vi "setControlAmplitude.vi"(8 "error in":errorcluster, 9 "amplitude":i32, 10 "axis":i32, 11 "connection ID":i32) -> (0 "error out":errorcluster, 2 "axis_out":i32, 3 "connection ID":i32)   [LabVIEW 2016]
doc: "This function sets the amplitude of the actuator signal of the selected axis."
panel:
  out "params_cluster":cluster{"axis":i32, "amplitude":i32}
  in  "Params_cluster":cluster{"integer":i32, "integer":i32}
  in  "results_cluster":cluster{"errNo":i32}
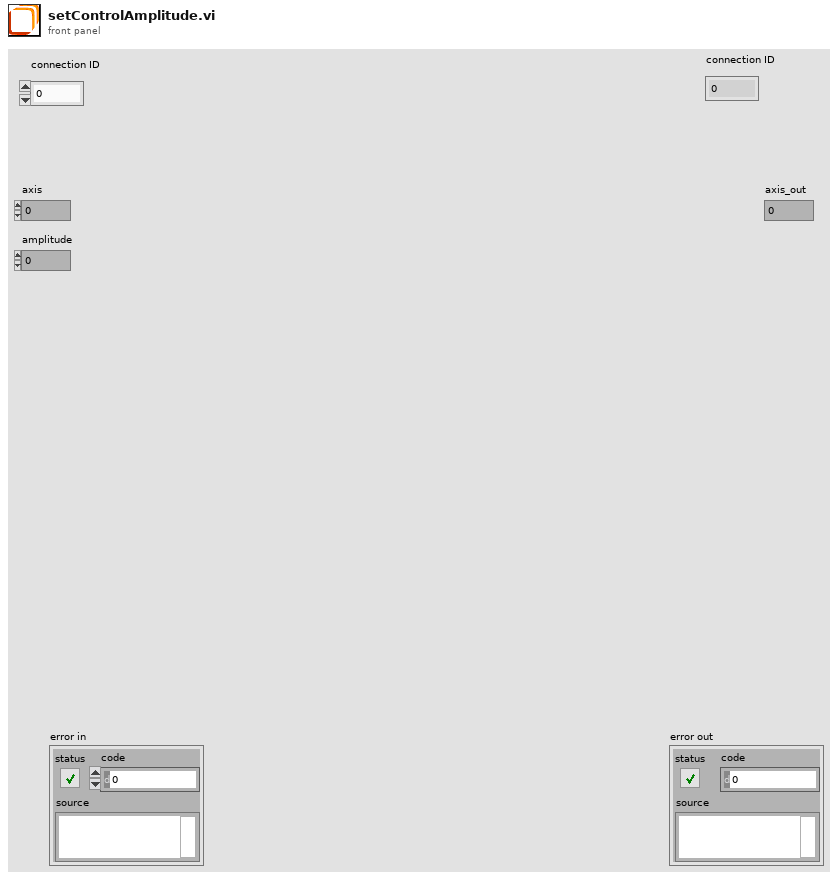
[diagram p1: front panel]
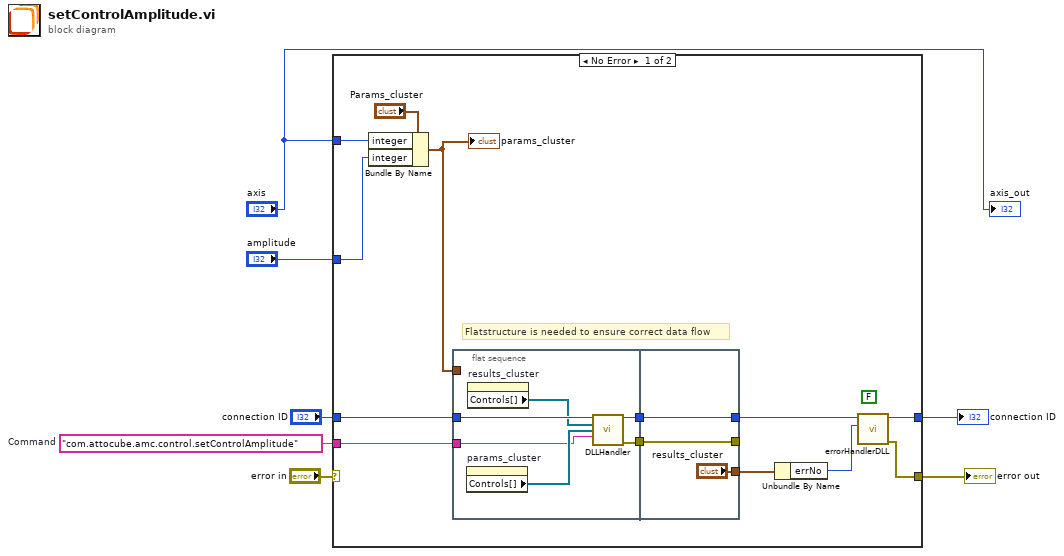
[diagram p0: block diagram]
diagram:
  w5 = "com.attocube.amc.control.setControlAmplitude"  # Command
  n1 = case shown="No Error" "error in" {
    selector: "error in" -> [_ w31]
    tunnel: [w10 w31] -> w7
    tunnel: "connection ID" -> [w20 w30]
    tunnel: w5 -> [w17 _]
    tunnel: [w12 w30] -> w3
    tunnel: "axis" -> [w9 _]
    tunnel: "amplitude" -> [w8 _]
    frame No Error {
      (unwired) FALSE ("show popup")
      # "Flatstructure is needed to ensure correct data flow"
      n2 = Bundle By Name(cluster="Params_cluster", "integer"=w9, "integer"=w8) -> (w15:cluster{"integer":i32, "integer":i32})
      "params_cluster" <- w15
      n3 = flat-sequence {
        tunnel: w20 -> [w26]
        tunnel: w17 -> [w23]
        tunnel: [w22] -> w16
        tunnel: w15 -> [_]
        tunnel: [w21] -> w13
        tunnel: ["results_cluster"] -> w19
        tunnel: [w29] -> w14
        tunnel: [w27] -> _
        tunnel: w16 -> [w27]
        tunnel: w13 -> [w29]
        frame #0 {
          n4 = property on="params_cluster" class="Clust (strict)"() -> ("Controls[]"=w24:refnum<vi>[])  [unwired: 2 in, 2 out]
          n5 = property on="results_cluster" class="Clust (strict)"() -> ("Controls[]"=w25:refnum<vi>[])  [unwired: 2 in, 2 out]
          n6 = call "DLLHandler.vi"("connection ID"=w26, "results_cluster"=w25, "params_cluster"=w24, "method"=w23) -> ("connection ID out"=w21:i32, "error"=w22:errorcluster)  [unwired: 10 in]
        }
        frame #1 {
        }
      }
      n7 = Unbundle By Name(w19) -> ("errNo"=w11:i32)
      n8 = call "errorHandlerDLL.vi"("error number"=w11, "connection ID"=w14) -> ("error out"=w10:errorcluster, "connection ID"=w12:i32)  [unwired: 8 in]
    }
    frame Error {
    }
  }
  "error out" <- w7
  "connection ID" <- w3
  "axis_out" <- "axis"
